vi "запис цифрових.vi"   [LabVIEW 2013]
uses:
  <vilib>/DAQmx/write.llb/DAQmx Write (Digital 1D Bool NChan 1Samp 1Line).vi
  <vilib>/DAQmx/write.llb/DAQmx Write (Digital Bool 1Line 1Point).vi
  <vilib>/DAQmx/create/channels.llb/DAQmx Create Channel (DO-Digital Output).vi
  <vilib>/DAQmx/miscellaneous.llb/DAQmx Fill In Error Info.vi
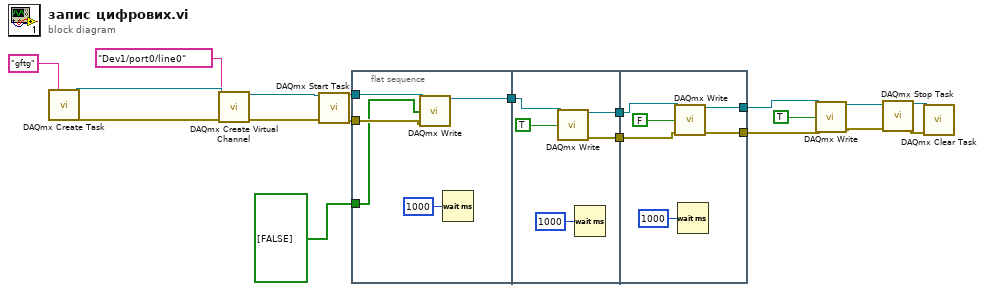
[diagram p0: block diagram]
diagram:
  n1 = call <vilib>:"DAQmx Create Task.vi"("new task name"="gftg") -> ("task out"=w18:refnum<k21>, "error out"=w16:errorcluster)  [unwired: 13 in]
  n2 = call-poly <vilib>:"DAQmx Create Virtual Channel.vi"("task in"=w18, "lines"=tag "Dev1/port0/line0", "error in"=w16) -> ("task out"=w15:refnum<k21>, "error out"=w14:errorcluster)  [unwired: 11 in]
  n3 = call <vilib>:"DAQmx Start Task.vi"("task/channels in"=w15, "error in"=w14) -> ("task out"=w13:refnum<k21>, "error out"=w8:errorcluster)  [unwired: 12 in]
  n4 = flat-sequence {
    tunnel: w13 -> [w24]
    tunnel: [w23] -> w11
    tunnel: w8 -> [w21]
    tunnel: bool[] [FALSE] ("data") -> [w20]
    tunnel: w11 -> [w28]
    tunnel: [w27] -> w10
    tunnel: [w25] -> w7
    tunnel: w10 -> [w34]
    tunnel: [w33] -> w9
    tunnel: w7 -> [w31]
    tunnel: [w30] -> w6
    frame #0 {
      n5 = call-poly <vilib>:"DAQmx Write.vi"("task/channels in"=w24, "data"=w20, "error in"=w21) -> ("task out"=w23:refnum<k21>)  [unwired: 10 in, 2 out]
      n6 = Wait (ms)(milliseconds to wait=u32 1000) -> ()  [unwired: 1 out]
    }
    frame #1 {
      n7 = call-poly <vilib>:"DAQmx Write.vi"("task/channels in"=w28, "data"=TRUE) -> ("task out"=w27:refnum<k21>, "error out"=w25:errorcluster)  [unwired: 11 in, 1 out]
      n8 = Wait (ms)(milliseconds to wait=u32 1000) -> ()  [unwired: 1 out]
    }
    frame #2 {
      n9 = call-poly <vilib>:"DAQmx Write.vi"("task/channels in"=w34, "data"=FALSE, "error in"=w31) -> ("task out"=w33:refnum<k21>, "error out"=w30:errorcluster)  [unwired: 10 in, 1 out]
      n10 = Wait (ms)(milliseconds to wait=u32 1000) -> ()  [unwired: 1 out]
    }
  }
  n11 = call-poly <vilib>:"DAQmx Write.vi"("task/channels in"=w9, "data"=TRUE, "error in"=w6) -> ("task out"=w5:refnum<k21>, "error out"=w2:errorcluster)  [unwired: 10 in, 1 out]
  n12 = call <vilib>:"DAQmx Stop Task.vi"("task/channels in"=w5, "error in"=w2) -> ("task out"=w4:refnum<k21>, "error out"=w3:errorcluster)  [unwired: 12 in]
  n13 = call <vilib>:"DAQmx Clear Task.vi"("task in"=w4, "error in"=w3) -> ()  [unwired: 13 in, 1 out]
